vi "OPC UA Client.vi"() -> ()   [LabVIEW 2018]
uses:
  <vilib>/OPCUA/controls/NodeIds.ctl
  <vilib>/OPCUA/controls/NodeId.ctl
  <vilib>/OPCUA/client/Multiple Read UInt64.vi
  <vilib>/OPCUA/NI OPC UA Client.lvlib
panel:
  out "Voltage":u64
  out "Frequency":u64
  in  "stop":bool
  out "error out":errorcluster
  in  "Server endpoint URL":string
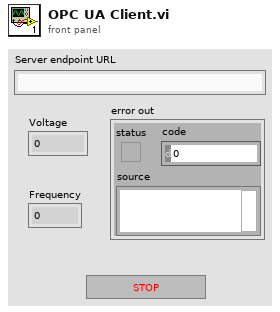
[diagram p1: front panel]
types:
  T1 = typedef "OPC UA Client Refnum.ctl" = refnum<k21>
  T2 = typedef "NodeIds.ctl" = T3[]
  T3 = typedef "NodeId.ctl" = string
  T4 = typedef "OPC UA StatusCode.ctl" = u32
  T5 = cluster{"node ID":T3, "value ":u64, "timestamp":timestamp, "status":T4}[]
  T6 = cluster{"node ID":T3, "value ":u64, "timestamp":timestamp, "status":T4}
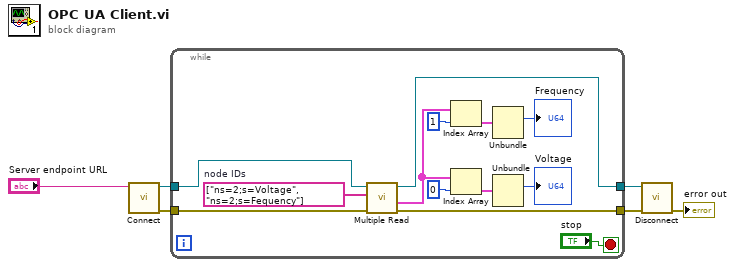
[diagram p0: block diagram]
diagram:
  n1 = call <vilib>:"Connect.vi"("server endpoint URL"="Server endpoint URL") -> ("error out"=w3:errorcluster, "OPC UA client refnum out"=w4:T1)  [unwired: 8 in, 1 out]
  n2 = while {
    tunnel: w4 -> [w17]
    tunnel: w3 -> [w16]
    tunnel: [w15] -> w2
    tunnel: [w14] -> w1
    stop <- "stop" stop-if-true
    w18 = T2 ["ns=2;s=Voltage", "ns=2;s=Fequency"]  # node IDs
    n3 = call-poly <vilib>:"Multiple Read.vi"("error in (no error)"=w16, "node IDs"=w18, "OPC UA client refnum in"=w17) -> ("error out"=w15:errorcluster, "results"=w10:T5, "OPC UA client refnum out"=w14:T1)  [unwired: 5 in, 1 out]
    n4 = Index Array(array=w10, index=1) -> (element=w13:T6)
    n5 = Index Array(array=w10, index=0) -> (element=w8:T6)
    n6 = Unbundle(w13) -> ("value"=→"Frequency":u64)  [unwired: 3 out]
    n7 = Unbundle(w8) -> ("value"=→"Voltage":u64)  [unwired: 3 out]
  }
  n8 = call <vilib>:"Disconnect.vi"("error in (no error)"=w2, "OPC UA client refnum in"=w1) -> ("error out"=→"error out":errorcluster)  [unwired: 9 in]
